vi "PH_Synchrolock_Watch.evt call Set Waveform End.vi"(0 "i ref in":refnum<vi>, 2 "Instance":string="N/A", 3 "Waveform End":i32=10000, 5 "error in (no error)":errorcluster) -> (14 "i ref out":refnum<vi>, 19 "error out":errorcluster)   [LabVIEW 2014, in "PH_Synchrolock_Watch.lvlib"]
doc: "This VI calls the \"SetTimebase\" case."
uses:
  PH_Synchrolock_Watch.lvlib
  CS_Core/CSSystem/CoreLib/CoreLib.int 2 byte array.vi
  CS_Core/CSSystem/CoreLib/CoreLib.lvlib
  CS_Core/BaseProcess/BaseProcess.lvlib
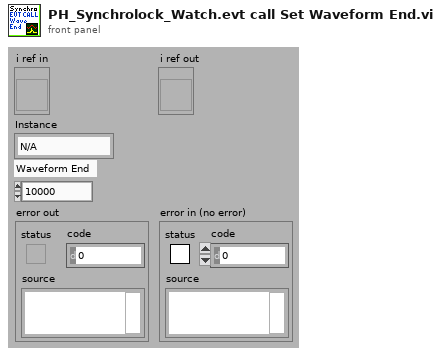
[diagram p1: front panel]
types:
  T1 = typedef "CoreDefs.rawDataType.ctl" = i8[]
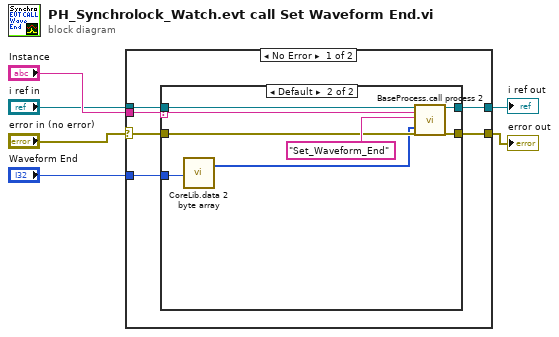
[diagram p0: block diagram]
diagram:
  n1 = case shown="No Error" "error in (no error)" {
    selector: "error in (no error)" -> [w8 w23]
    tunnel: [w12 w24] -> w3
    tunnel: [w11 w23] -> w2
    tunnel: "i ref in" -> [w10 w24]
    tunnel: "Waveform End" -> [w7 _]
    tunnel: "Instance" -> [w9 _]
    frame No Error {
      n2 = case shown="Default" w9 {
        selector: w9 -> [_ w17]
        tunnel: [w13 w21] -> w12
        tunnel: [w14 w20] -> w11
        tunnel: w10 -> [w13 w19]
        tunnel: w8 -> [w14 w18]
        tunnel: w7 -> [_ w16]
        frame "N/A" {
        }
        frame Default {
          n3 = call-poly "CoreLib.data 2 byte array.vi"("i32"=w16) -> ("byteArray out"=w15:T1)  [unwired: 18 in]
          n4 = call "BaseProcess.call process 2.vi"("i ref in"=w19, "Object"=w17, "Selector"="Set_Waveform_End", "Data"=w15, "error in (no error)"=w18) -> ("i ref out"=w21:refnum<vi>, "error out"=w20:errorcluster)  [unwired: 13 in]
        }
      }
    }
    frame Error {
    }
  }
  "error out" <- w2
  "i ref out" <- w3
